vi "簇案例之学生账号密码查询.vi"() -> ()   [LabVIEW 2018]
panel:
  out "簇 2":cluster{"学号":string, "密码":string, "是否缴费":bool}
  in  "簇":T1
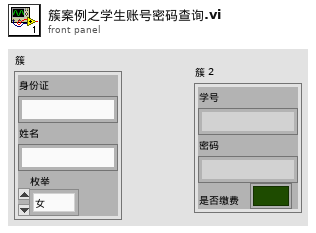
[diagram p1: front panel]
types:
  T1 = cluster{"身份证":string, "姓名":string, "枚举":enum16{"女", "男"}}
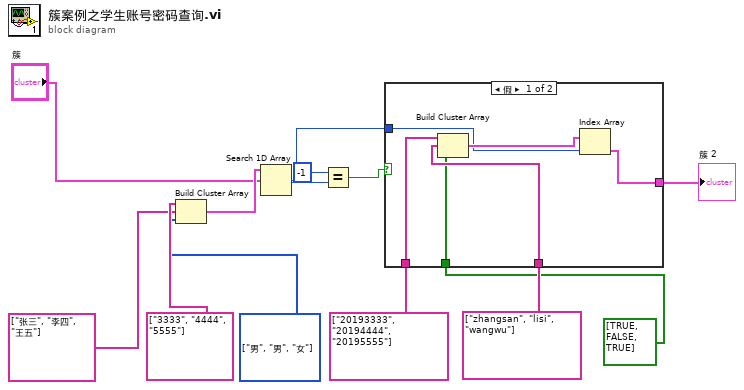
[diagram p0: block diagram]
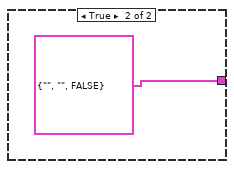
[diagram p2: hidden frame]
diagram:
  w10 = enum16{"女", "男"}[] [enum."男", enum."男", enum."女"] items=["女", "男"]
  n1 = Build Cluster Array(string[] ["3333", "4444", "5555"], string[] ["张三", "李四", "王五"], w10) -> (w9:cluster{string, string, enum16{"女", "男"}}[])
  n2 = Search 1D Array(1D array=w9, element="簇") -> (index of element=w1:i32)  [unwired: 1 in]
  n3 = Equal?(x=-1, y=w1) -> (x = y?=w6:bool)
  n4 = case shown="假" w6 {
    tunnel: [w13 cluster{string, string, bool} {"", "", FALSE}] -> w5
    tunnel: string[] ["20193333", "20194444", "20195555"] -> [w18 _]
    tunnel: string[] ["zhangsan", "lisi", "wangwu"] -> [w17 _]
    tunnel: bool[] [TRUE, FALSE, TRUE] -> [w16 _]
    tunnel: w1 -> [w14 _]
    frame False {
      n5 = Build Cluster Array(w18, w17, w16) -> (w15:cluster{string, string, bool}[])
      n6 = Index Array(array=w15, index=w14) -> (element=w13:cluster{string, string, bool})
    }
    frame True {
    }
  }
  "簇 2" <- w5
